vi "Intake Execute.vi"   [LabVIEW 2016]
uses:
  Intake Control Type.ctl
  <vilib>/Rock Robotics/WPI/DriverStation/WPI_DriverStationRobotMode2.ctl
  Intake Notifier.ctl
  Intake Globals.vi
  Robot Global Data.vi
types:
  T1 = typedef "WPI_MotorControlDeviceRef.ctl" = cluster{"DeviceStatus":errorcluster, "Type":T2, "PWM":cluster{"PWM Channel":T3, "DeadBand":T4}, "CAN":cluster{"Device Number":u8, "SetOutput VI Ref":variant, "GetOutput VI Ref":variant, "Enable VI Ref":variant, "Disable VI Ref":variant, "Data":variant}, "Invert":bool}
  T2 = typedef "WPI_MotorControlType.ctl" = enum16{"PWM", "CAN"}
  T3 = typedef "FPGA_DIOPWMChannel.ctl" = enum8{"PWM 0", "PWM 1", "PWM 2", "PWM 3", "PWM 4", "PWM 5", "PWM 6", "PWM 7", "PWM 8", "PWM 9", "PWM MXP 0", "PWM MXP 1", "PWM MXP 2", "PWM MXP 3", "PWM MXP 4", "PWM MXP 5", "PWM MXP 6", "PWM MXP 7", "PWM MXP 8", "PWM MXP 9", "Invalid"}
  T4 = typedef "WPI_PWMDeadband.ctl" = cluster{"Name":string, "maxPositivePwm":i32, "minPositivePwm":i32, "centerPwm":i32, "maxNegativePwm":i32, "minNegativePwm":i32, "angularRange":u16}
  T5 = typedef "Intake Control Type.ctl" = enum16{"No Op", "In", "Out"}
  T6 = typedef "Intake Notifier.ctl" = cluster{"In":bool, "Out":bool, "Intake Control List":T5, "Parameter 1":dbl, "Parameter 2":dbl, "Intake Notifier":refnum<notifier>, "Step":i32}
  T7 = typedef "WPI_DriverStationRobotMode2.ctl" = enum16{"Autonomous Disabled", "Autonomous Enabled", "Teleop Disabled", "Teleop Enabled", "Disconnected", "Finish", "Test Disabled", "Test Enabled", "Emergency Stopped"}
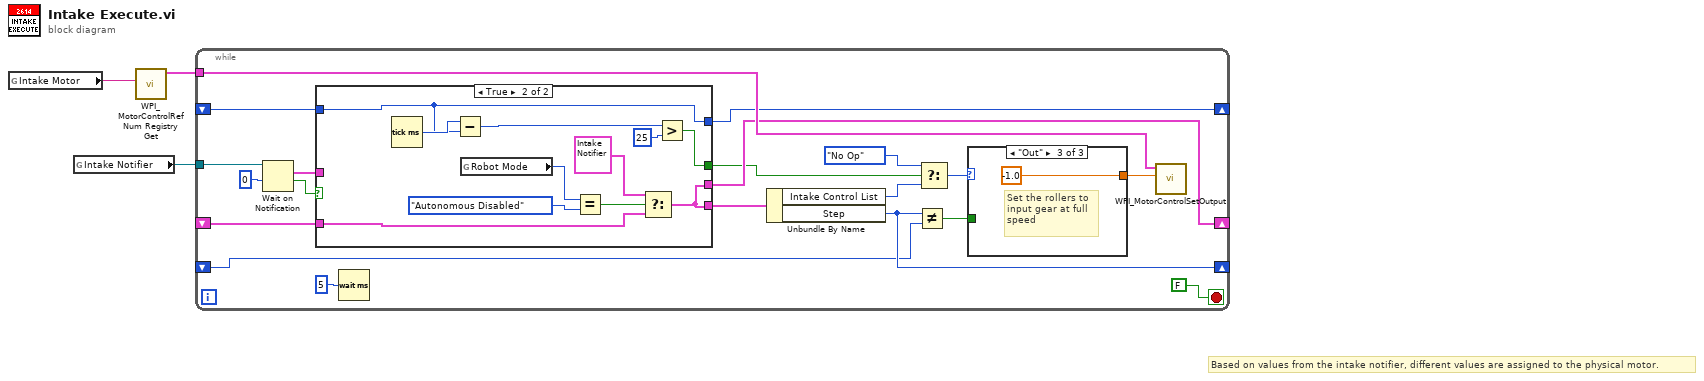
[diagram p0: block diagram]
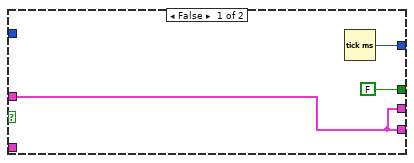
[diagram p2: hidden frame]
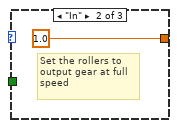
[diagram p4: hidden frame]
diagram:
  # "Based on values from the intake notifier, different values are assigned to the physical motor."
  n1 = global read "Intake Globals.vi" "Intake Motor"() -> (w1:string)
  n2 = global read "Intake Globals.vi" "Intake Notifier"() -> (w3:refnum<notifier>)
  n3 = call <vilib>:"WPI_MotorControlRefNum Registry Get.vi"("refnum name"=w1) -> ("MotorControlDevRef"=w2:T1)  [unwired: 9 in, 1 out]
  n4 = while {
    tunnel: w3 -> [w21]
    tunnel: w2 -> [w20]
    shift-right: [w16] -> _
    shift-left: _ -> [w15]
    shift-right: [w12] -> _
    shift-left: _ -> [w7]
    shift-right: [w5] -> _
    shift-left: _ -> [w4]
    stop <- FALSE stop-if-true
    n5 = Wait on Notification(notifier=w21, timeout in ms (-1)=0) -> (notification=w14:T6, timed out?=w17:bool)  [unwired: 2 in, 2 out]
    n6 = case shown="True" w17 {
      tunnel: w14 -> [w26 _]
      tunnel: [w26 w27] -> w12
      tunnel: [w26 w27] -> w13
      tunnel: [w25 w36] -> w16
      tunnel: w15 -> [_ w36]
      tunnel: [FALSE w33] -> w11
      tunnel: w7 -> [_ w29]
      frame False {
        n7 = Tick Count (ms)() -> (millisecond timer value=w25:u32)
      }
      frame True {
        n8 = Tick Count (ms)() -> (millisecond timer value=w37:u32)
        n9 = Subtract(x=w37, y=w36) -> (x-y=w35:u32)
        n10 = global read "Robot Global Data.vi" "Robot Mode"() -> (w32:T7)
        n11 = Equal?(x=w32, y=WPI_DriverStationRobotMode2."Autonomous Disabled") -> (x = y?=w30:bool)
        n12 = Select(t=T6 {"In"=FALSE, "Out"=FALSE, "Intake Control List"=enum."No Op", "Parameter 1"=0.0, "Parameter 2"=0.0, "Intake Notifier"=refnum, "Step"=0} ("Intake Notifier"), s=w30, f=w29) -> (s? t:f=w27:T6)
        n13 = Greater?(x=w35, y=u32 25) -> (0:w33:bool)
      }
    }
    n14 = Wait (ms)(milliseconds to wait=u32 5) -> ()  [unwired: 1 out]
    n15 = Unbundle By Name(w13) -> ("Intake Control List"=w10:T5, "Step"=w5:i32)
    n16 = Not Equal?(x=w5, y=w4) -> (x != y?=w6:bool)
    n17 = Select(t=Intake_Control_Type."No Op", s=w11, f=w10) -> (s? t:f=w9:T5)
    n18 = case shown="\"Out\"" w9 {
      tunnel: [_ 1.0 ("Output") -1.0 ("Output")] -> w19
      tunnel: w6 -> [_ _ _]
      frame "No Op", Default {
      }
      frame "In" {
        # "Set the rollers to \noutput gear at full \nspeed"
      }
      frame "Out" {
        # "Set the rollers to \ninput gear at full \nspeed"
      }
    }
    n19 = call <vilib>:"WPI_MotorControlSetOutput.vi"("Output"=w19, "MotorControlDevRef"=w20) -> ()  [unwired: 7 in, 3 out]
  }
